vi "Read Instr CFGs.vi"(8 "error in":errorcluster, 10 "Series Id":u32, 11 "Database UI in":refnum<class "Database UI.lvclass">) -> (0 "error out":errorcluster, 3 "Database UI out":refnum<class "Database UI.lvclass">)   [LabVIEW 2023, in "Database UI.lvlib" / "Database UI.lvclass"]
uses:
  Database UI.lvclass
  Database UI.lvclass/Database UI.ctl
  <vilib>/drjdpowell/SQLite Library/SQL Statement/SQL Statement.lvclass/SQL Statement.ctl
  <vilib>/drjdpowell/SQLite Library/SQL Statement/Get Column Names.vi
  <vilib>/drjdpowell/SQLite Library/SQL Statement/Get Column Count.vi
  <vilib>/drjdpowell/SQLite Library/SQL Statement/Write Next Column.vi
  <vilib>/drjdpowell/SQLite Library/SQL Statement/Get Column Name.vi
  <vilib>/drjdpowell/SQLite Library/SQL Statement/Error Message.vi
  <vilib>/drjdpowell/SQLite Library/SQL Statement/Column String.vi
  <vilib>/drjdpowell/SQLite Library/SQL Connection/Connection.lvclass
  <vilib>/drjdpowell/SQLite Library/SQL Statement/SQL Statement.lvclass
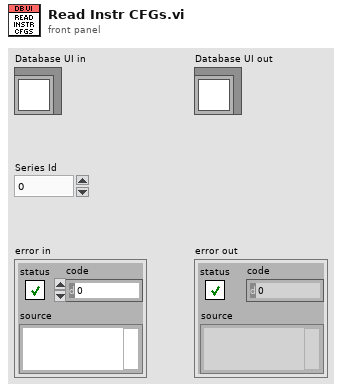
[diagram p1: front panel]
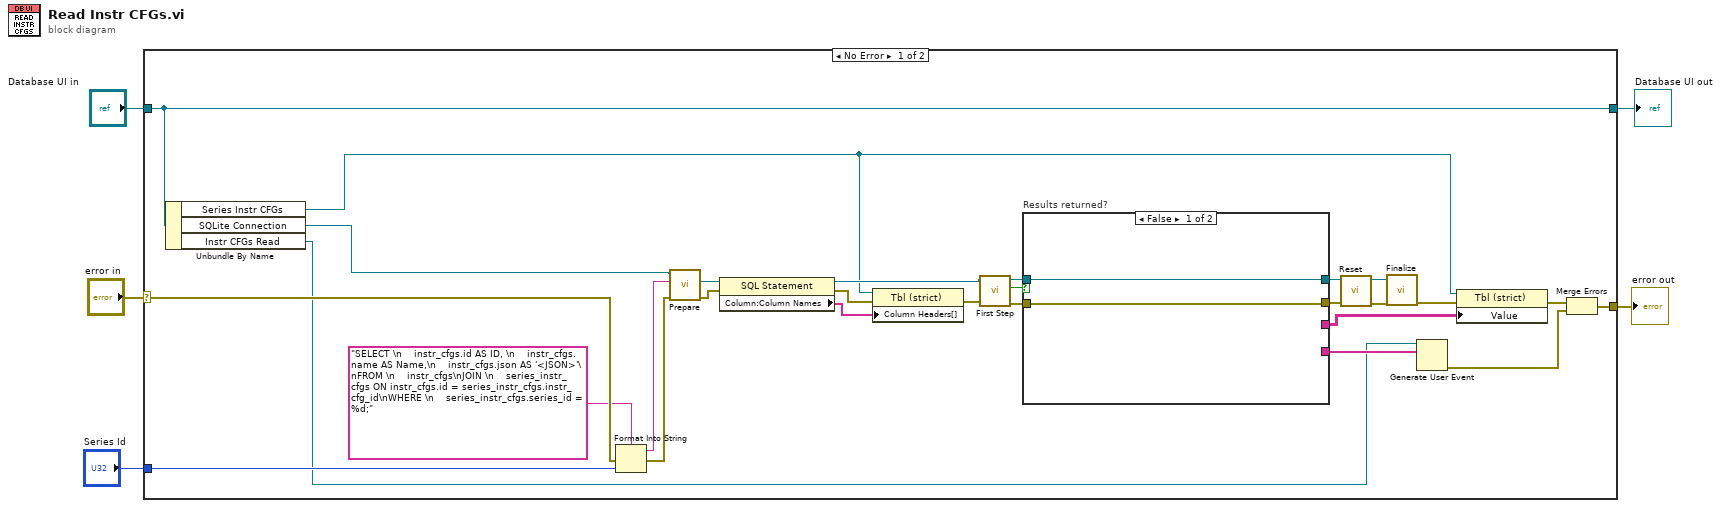
[diagram p0: block diagram]
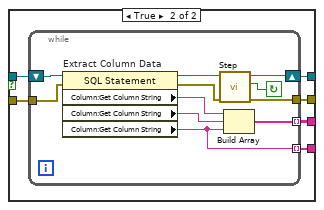
[diagram p2: hidden frame]
diagram:
  n1 = case shown="No Error" "error in" {
    selector: "error in" -> [w23 w54]
    tunnel: [w8 w54] -> w4
    tunnel: [w11 w53] -> w2
    tunnel: "Database UI in" -> [w11 w53]
    tunnel: "Series Id" -> [w21 _]
    frame No Error {
      n2 = Unbundle By Name(w11) -> ("Series Instr CFGs"=w25:refnum<vi>, "SQLite Connection"=w6:refnum<class "Connection.lvclass">, "Instr CFGs Read"=w9:refnum<user-event>)
      n3 = Format Into String(format string="SELECT \n    instr_cfgs.id AS ID, \n    instr_cfgs.name AS Name,\n    instr_cfgs.json AS '<JSON>'\nFROM \n    instr_cfgs\nJOIN \n    series_instr_cfgs ON instr_cfgs.id = series_instr_cfgs.instr_cfg_id\nWHERE \n    series_instr_cfgs.series_id = %d;", error in=w23, w21) -> (resulting string=w19:string, error out=w20:errorcluster)  [unwired: 1 in]
      n4 = call <vilib>:"Prepare.vi"("error in (no error)"=w20, "SQL"=w19, "SQLite Connection in"=w6) -> ("error out"=w32:errorcluster, "SQL Statement"=w33:refnum<class "SQL Statement.lvclass">)  [unwired: 4 in, 3 out]
      n5 = property class="SQL Statement"(reference=w33, error in=w32) -> (reference out=w28:refnum<class "SQL Statement.lvclass">, error out=w30:errorcluster, "Column:Column Names"=w31:string[])
      n6 = property on="Property Node" class="Tbl (strict)"(reference=w25, error in=w30, "Column Headers[]"=w31) -> (error out=w29:errorcluster)  [unwired: 1 out]
      n7 = call <vilib>:"First Step.vi"("error in (no error)"=w29, "SQL Statement in"=w28) -> ("error out"=w16:errorcluster, "Row returned"=w12:bool, "SQL Statement"=w17:refnum<class "SQL Statement.lvclass">)  [unwired: 7 in]
      n8 = case "Results returned?" shown="False" w12 {
        tunnel: w17 -> [w34 w41]
        tunnel: w16 -> [w35 w40]
        tunnel: [w35 w39] -> w14
        tunnel: [w34 w38] -> w15
        tunnel: [_ w37] -> w13
        tunnel: [_ w36] -> w10
        frame False {
        }
        frame True {
          n9 = while {
            shift-right: [w49] -> w38
            shift-left: w41 -> [w52]
            tunnel: w40 -> [w50]
            tunnel: [w46] -> w39
            tunnel: [w43] -> w37 mode=indexing
            tunnel: [w42] -> w36 mode=indexing
            stop <- w47 continue-if-true
            n10 = property on="Extract Column Data" class="SQL Statement"(reference=w52, error in=w50) -> (reference out=w51:refnum<class "SQL Statement.lvclass">, error out=w48:errorcluster, "Column:Get Column String"=w45:string, "Column:Get Column String"=w44:string, "Column:Get Column String"=w42:string)
            n11 = call <vilib>:"Step.vi"("error in (no error)"=w48, "SQL Statement in"=w51) -> ("error out"=w46:errorcluster, "Row returned"=w47:bool, "SQL Statement"=w49:refnum<class "SQL Statement.lvclass">)  [unwired: 7 in]
            n12 = Build Array(w45, w44, w42) -> (w43:string[])
          }
        }
      }
      n13 = call <vilib>:"Reset.vi"("error in (no error)"=w14, "SQL Statement in"=w15) -> ("error out"=w26:errorcluster, "SQL Statement"=w27:refnum<class "SQL Statement.lvclass">)  [unwired: 8 in]
      n14 = call <vilib>:"Finalize.vi"("error in (no error)"=w26, "SQL Statement in"=w27) -> ("error out"=w24:errorcluster)  [unwired: 9 in]
      n15 = Generate User Event(user event=w9, event data cluster=w10) -> (error out=w7:errorcluster)  [unwired: 2 in, 1 out]
      n16 = property class="Tbl (strict)"(reference=w25, error in=w24, "Value"=w13) -> (error out=w18:errorcluster)  [unwired: 1 out]
      n17 = Merge Errors(w18, w7) -> (w8:errorcluster)
    }
    frame Error {
    }
  }
  "error out" <- w4
  "Database UI out" <- w2
